vi "Senado.vi"() -> ()   [LabVIEW 2017]
uses:
  <vilib>/Simulation/Scripting/Companion Diagram/SimConfigNode/SimParams.ctl
  <vilib>/Simulation/Scripting/Companion Diagram/SimConfigNode/_simSolvers.ctl
  <vilib>/Simulation/Implementation/Shared/SIMSCR Execution Mode.ctl
  <vilib>/Simulation/Param Hierarchy/Typedefs/SIMPH Param Control Actions.ctl
  <vilib>/Simulation/Implementation/Shared/NILVSim_ParamChanged.vi
  <vilib>/Simulation/Implementation/Shared/NILVSIM_BeginStep.vi
  <vilib>/Simulation/DataSources/Implementation/NILVSim Step.llb/SIM Step (scalar).vi
  <vilib>/Simulation/Utility/Implementation/SIM Halt.vi
  <vilib>/Simulation/ContinuousLinear/Implementation/NILVSim Transfer Function.llb/SIM Transfer Function Distributor (SISO).vi
  <vilib>/Simulation/ContinuousLinear/Implementation/NILVSim Transfer Function.llb/SIM Transfer Function Collector (SISO).vi
  <vilib>/Simulation/SignalDisplay/Implementation/NILVSim Time Waveform.llb/SIM Time Waveform (scalar).vi
  <vilib>/Simulation/Implementation/Shared/NILVSim_Manager.vi
  <vilib>/Utility/error.llb/Clear Errors.vi
  <vilib>/Simulation/Implementation/Shared/NILVSim_FinalizeModel.vi
  <vilib>/picture/3D Picture Control/Object/Create Object (drawable).vi
  <vilib>/Simulation/Implementation/Shared/SIM Unbundle Sim Info.vi
  <vilib>/Simulation/Implementation/Shared/NILVSim_Initialize.vi
  <vilib>/picture/3D Picture Control/Transformations/Set Translation.vi
  <vilib>/picture/3D Picture Control/Object/Add Object.vi
  <vilib>/picture/3D Picture Control/Object/Add Object (reference).vi
  <vilib>/Simulation/Utility/Implementation/NILVSim Get Time and IsAcceptedStep.vi
  <vilib>/Simulation/Implementation/Shared/SIMSH Read Queue.vi
  <vilib>/Simulation/Implementation/Shared/NILVSim_GetModelError.vi
  <vilib>/Simulation/Implementation/Shared/SIM Bundle Sim Info.vi
  <vilib>/Simulation/Scripting/Companion Diagram/SimConfigNode/SimDog.xnode
  <vilib>/Simulation/Implementation/XNodeFramework/SimXNode/SimX.xnode
  <vilib>/picture/3D Picture Control/NI_3D Picture Control.lvlib
  <vilib>/Simulation/ContinuousLinear/Implementation/NILVSim Transfer Function.llb/SIM Transfer Function (SISO).vi
  <vilib>/Simulation/Implementation/Shared/NI_SIM_Implementation.lvlib
panel:
  out "3D Picture":refnum<vi>(3d-picture)
  in  "Halt?":bool
  out "Waveform Chart":waveform(dbl)(graph)
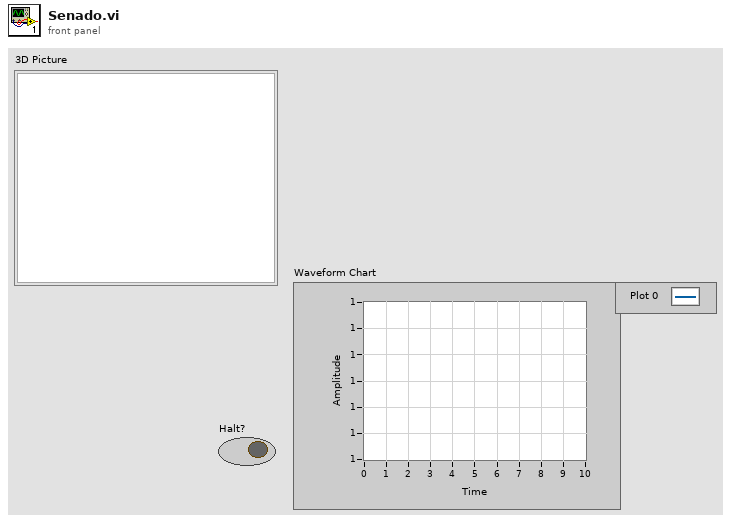
[diagram p1: front panel]
types:
  T1 = cluster{"Red":sgl, "Green":sgl, "Blue":sgl, "Alpha":sgl}
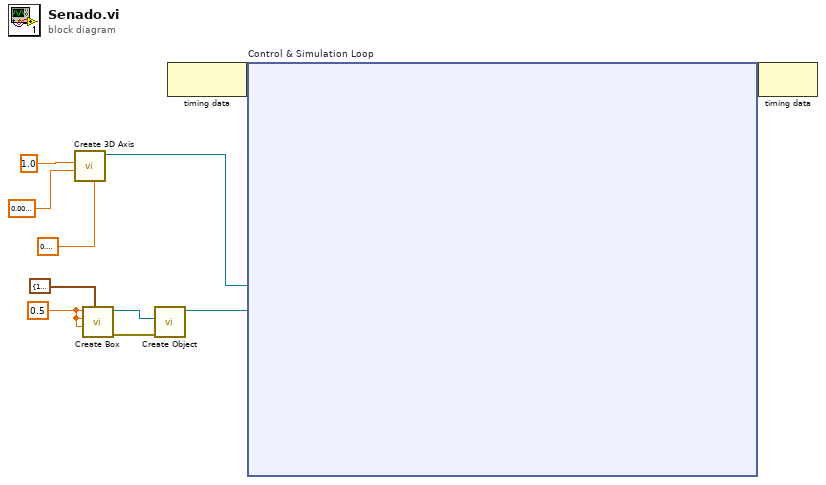
[diagram p0: block diagram]
diagram:
  w8 = sgl 0.5 ("Length X")
  n1 = call <vilib>:"Create 3D Axis.vi"("Character Size"=sgl 0.1, "Radius"=sgl 0.01, "Length"=sgl 1.0) -> ("New Object Refnum"=w1:refnum<vi>)  [unwired: 7 in, 1 out]
  n2 = call <vilib>:"Create Box.vi"("Color"=T1 {"Red"=1.0, "Green"=0.0, "Blue"=0.0, "Alpha"=1.0}, "Length Z"=w8, "Length Y"=w8, "Length X"=w8) -> ("error out"=w7:errorcluster, "New Box Refnum"=w6:refnum<vi>)  [unwired: 6 in]
  n3 = call-poly <vilib>:"Create Object.vi"("error in (no error)"=w7, "Geometry"=w6) -> ("Scene:New Object"=w5:refnum<vi>)  [unwired: 8 in, 1 out]
  n4 = node-c288() -> (w11:variant)  [unwired: 1 in]
  n5 = node-c254 "Control & Simulation Loop"(w11, w5, w1) -> (w10:variant)  [unwired: 1 out]
  n6 = node-c288(w10) -> ()  [unwired: 1 out]
